vi "Configure Clock Source.vi"(8 "error in (no error)":errorcluster, 9 "Source (0: Internal)":u16(ring) items=["Internal", "External", "TTL", "0V"], 10 "Type Of Clock (0: Reference Clock)":u16(ring) items=["Reference Clock", "Sample Clock"], 11 "VISA resource name":refnum<visa-resource-name>) -> (0 "error out":errorcluster, 3 "VISA resource name out":refnum<visa-resource-name>)   [LabVIEW 2015, in "LeCroy Wave Series.lvlib"]
doc: "Toggles between internal clock and external clock for reference clock and sample clock."
uses:
  <instrlib>/LeCroy Wave Series/LeCroy Wave Series.lvlib
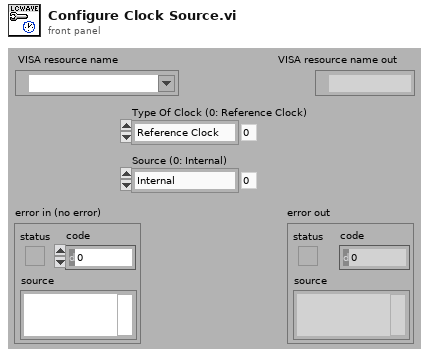
[diagram p1: front panel]
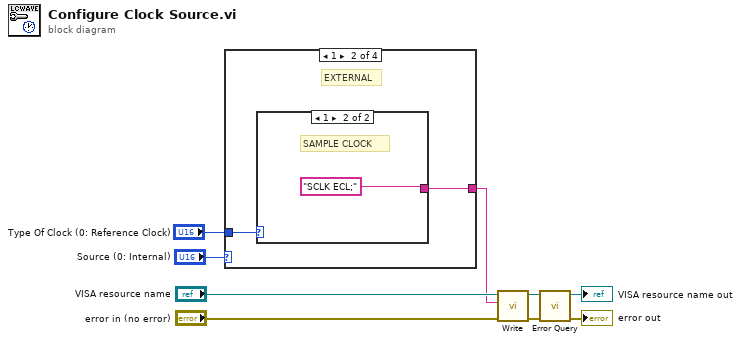
[diagram p0: block diagram]
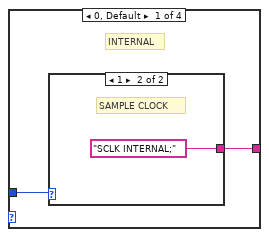
[diagram p2: hidden frame]
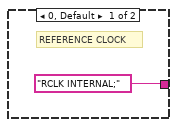
[diagram p3: hidden frame]
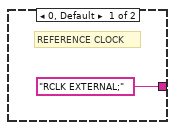
[diagram p4: hidden frame]
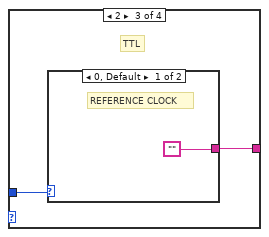
[diagram p5: hidden frame]
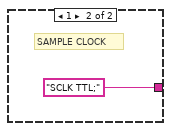
[diagram p6: hidden frame]
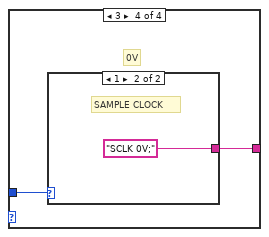
[diagram p7: hidden frame]
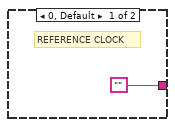
[diagram p8: hidden frame]
diagram:
  n1 = case shown="1" "Source (0: Internal)" {
    tunnel: "Type Of Clock (0: Reference Clock)" -> [w11 w15 w19 w23]
    tunnel: [w10 w14 w18 w22] -> w1
    frame 0, Default {
      # "INTERNAL"
      n2 = case shown="1" w11 {
        tunnel: ["RCLK INTERNAL;" "SCLK INTERNAL;"] -> w10
        frame 0, Default {
          # "REFERENCE CLOCK"
        }
        frame 1 {
          # "SAMPLE CLOCK"
        }
      }
    }
    frame 1 {
      # "EXTERNAL"
      n3 = case shown="1" w15 {
        tunnel: ["RCLK EXTERNAL;" "SCLK ECL;"] -> w14
        frame 0, Default {
          # "REFERENCE CLOCK"
        }
        frame 1 {
          # "SAMPLE CLOCK"
        }
      }
    }
    frame 2 {
      # "TTL"
      n4 = case shown="0, Default" w19 {
        tunnel: ["" ("Empty String Constant") "SCLK TTL;"] -> w18
        frame 0, Default {
          # "REFERENCE CLOCK"
        }
        frame 1 {
          # "SAMPLE CLOCK"
        }
      }
    }
    frame 3 {
      # "0V"
      n5 = case shown="1" w23 {
        tunnel: ["" ("Empty String Constant") "SCLK 0V;"] -> w22
        frame 0, Default {
          # "REFERENCE CLOCK"
        }
        frame 1 {
          # "SAMPLE CLOCK"
        }
      }
    }
  }
  n6 = call <instrlib>:"Write.vi"("error in (no error)"="error in (no error)", "Write Buffer"=w1, "VISA resource name"="VISA resource name") -> ("error out"=w4:errorcluster, "VISA resource name out"=w5:refnum<visa-resource-name>)  [unwired: 6 in, 1 out]
  n7 = call <instrlib>:"Error Query.vi"("error in (no error)"=w4, "VISA resource name"=w5) -> ("error out"=→"error out":errorcluster, "VISA resource name out"=→"VISA resource name out":refnum<visa-resource-name>)  [unwired: 6 in, 2 out]
